vi "Activate Menu.vi"(7 "Coords":T1, 8 "error in":errorcluster, 9 "Menu Ref":refnum<k9>, 10 "Control Ref":refnum<vi>, 11 "Peer Review":refnum<class "Peer Review.lvclass">) -> (0 "error out":errorcluster, 2 "Discard?":bool)   [LabVIEW 2020, in "Peer Review.lvclass"]
uses:
  Peer Review.lvclass
  <vilib>/Utility/miscctls.llb/LVPoint32TypeDef.ctl
  Peer Review.lvclass/Peer Review.ctl
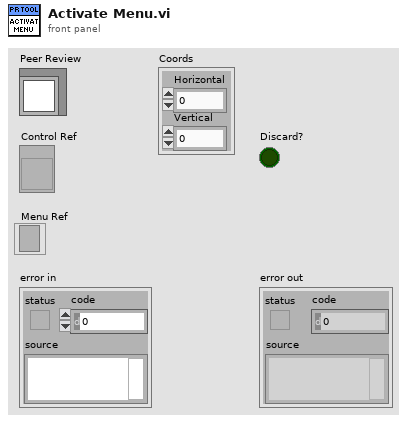
[diagram p1: front panel]
types:
  T1 = typedef "LVPoint32TypeDef.ctl" = cluster{"Horizontal":i32, "Vertical":i32}
  T2 = typedef "LVRowAndColumnTypeDef.ctl" = cluster{"Row":i32, "Column":i32}
  T3 = typedef "Peer Review.lvclass/File Info.ctl" = cluster{"File ID":i32, "Commit ID":i32, "Reviewed Hash":string, "Relative Path":string, "File Path":path, "File Checksum":string, "State":T4, "FP Changes":i32, "BD Changes":i32, "FP Bounds Error":dbl, "BD Bounds Error":dbl, "Lines Added":i32, "Lines Removed":i32, "Analysis Passes":i32, "Analysis Fails":i32, "Attribute Changes":i32, "Reentrancy Changes":string, "Cyclomatic Complexity":i32, "Node Count":i32, "Revision Number":u32, "LabVIEW Version":string, "Description":string, "Master Path":path, "Master Checksum":string, "VI Type":T5, "LabVIEW File":bool, "Review Complete":bool, "File Ref":refnum<vi>}
  T4 = typedef "Peer Review.lvclass/File State.ctl" = enum16{"Interrogation Needed", "Modified", "Deleted", "Added", "Matches Previous", "No Changes", "Moved"}
  T5 = typedef "Peer Review.lvclass/VI Type.ctl" = enum32{"invalid VI type", "Standard VI", "Control VI", "Global VI", "Polymorphic VI", "Configuration VI", "SubSystem", "Facade VI", "Method VI", "Statechart Diagram VI"}
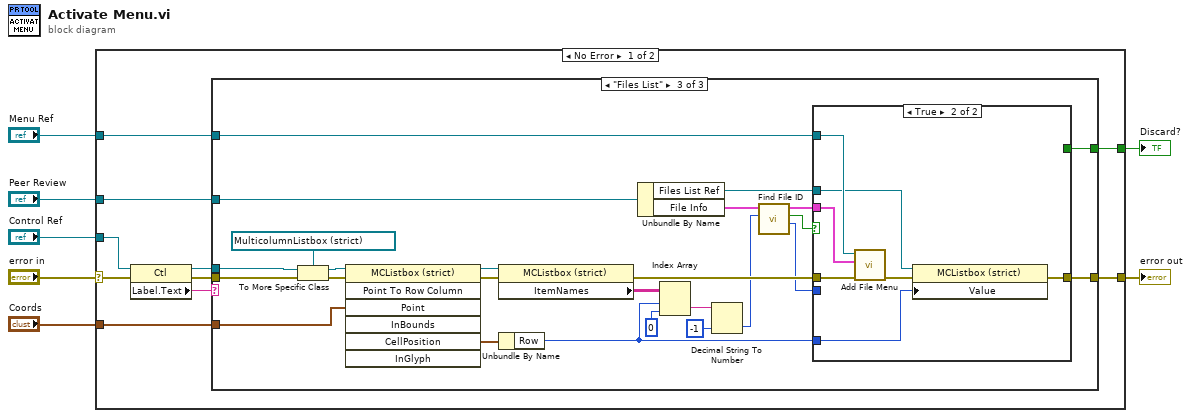
[diagram p0: block diagram]
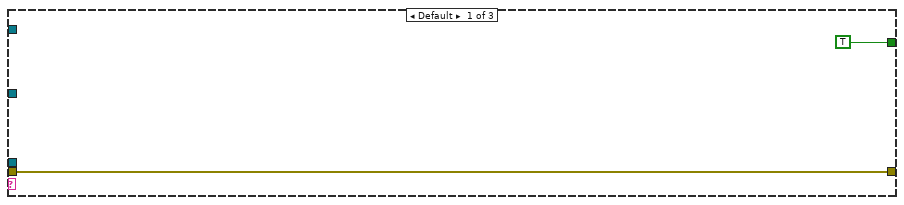
[diagram p2: hidden frame]
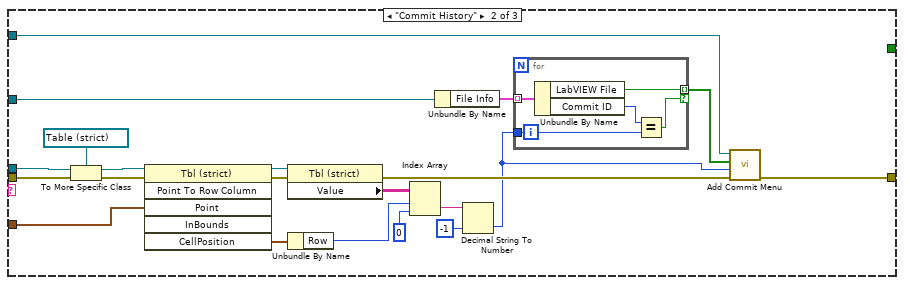
[diagram p3: hidden frame]
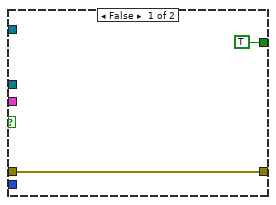
[diagram p4: hidden frame]
diagram:
  n1 = case shown="No Error" "error in" {
    selector: "error in" -> [w16 w80]
    tunnel: "Control Ref" -> [w17 _]
    tunnel: "Coords" -> [w13 _]
    tunnel: "Menu Ref" -> [w11 _]
    tunnel: [w10 w80] -> w3
    tunnel: [w9 _] -> w2
    tunnel: "Peer Review" -> [w8 _]
    frame No Error {
      n2 = property class="Ctl"(reference=w17, error in=w16) -> (reference out=w14:refnum<vi>, error out=w15:errorcluster, "Label.Text"=w12:string)
      n3 = case shown="\"Files List\"" w12 {
        tunnel: w15 -> [w19 w39 w70]
        tunnel: w14 -> [_ w38 w69]
        tunnel: w13 -> [_ w37 w68]
        tunnel: w11 -> [_ w34 w65]
        tunnel: [w19 w33 w64] -> w10
        tunnel: [TRUE _ w63] -> w9
        tunnel: w8 -> [_ w25 w55]
        frame Default {
        }
        frame "Commit History" {
          n4 = To More Specific Class(target class=refnum<vi> refnum ("Commit History Ref"), reference=w38, error in=w39) -> (specific class reference=w29:refnum<vi>, error out=w30:errorcluster)
          n5 = invoke class="Tbl (strict)" method="Point To Row Column"(reference=w29, error in=w30, "Point"=w37) -> (reference out=w27:refnum<vi>, error out=w26:errorcluster, "CellPosition"=w28:T2)  [unwired: 3 in, 3 out]
          n6 = property class="Tbl (strict)"(reference=w27, error in=w26) -> (error out=w35:errorcluster, "Value"=w36:string[][])  [unwired: 1 out]
          n7 = Unbundle By Name(w28) -> ("Row"=w40:i32)
          n8 = Index Array(array=w36, index (row)=w40, index (col)=0 ("disabled index (col)")) -> (element=w20:string)
          n9 = Unbundle By Name(w25) -> ("File Info"=w32:T3[])
          n10 = Decimal String To Number(string=w20, default (0L)=-1 ("default (0 I32)")) -> (number=w22:i32)  [unwired: 1 in, 1 out]
          n11 = for {
            tunnel: w32 -> [w44] mode=indexing
            tunnel: w22 -> [w45]
            tunnel: [w41] -> w23 mode=indexing if=w42
            n12 = Unbundle By Name(w44) -> ("LabVIEW File"=w41:bool, "Commit ID"=w43:i32)
            n13 = Equal?(x=w43, y=w45) -> (x = y?=w42:bool)
          }
          n14 = call "Add Commit Menu.vi"("error in"=w35, "Commit ID"=w22, "LabVIEW Files?"=w23, "Menu Ref"=w34) -> ("error out"=w33:errorcluster)  [unwired: 7 in]
        }
        frame "Files List" {
          n15 = To More Specific Class(target class=refnum<vi> refnum ("Files List Ref"), reference=w69, error in=w70) -> (specific class reference=w59:refnum<vi>, error out=w60:errorcluster)
          n16 = invoke class="MCListbox (strict)" method="Point To Row Column"(reference=w59, error in=w60, "Point"=w68) -> (reference out=w57:refnum<vi>, error out=w56:errorcluster, "CellPosition"=w58:T2)  [unwired: 4 in, 4 out]
          n17 = property class="MCListbox (strict)"(reference=w57, error in=w56) -> (error out=w66:errorcluster, "ItemNames"=w67:string[][])  [unwired: 1 out]
          n18 = Unbundle By Name(w58) -> ("Row"=w46:i32)
          n19 = Unbundle By Name(w55) -> ("Files List Ref"=w48:refnum<vi>, "File Info"=w52:T3[])
          n20 = Index Array(array=w67, index (row)=w46, index (col)=0 ("disabled index (col)")) -> (element=w53:string)
          n21 = Decimal String To Number(string=w53, default (0L)=-1 ("default (0 I32)")) -> (number=w51:i32)  [unwired: 1 in, 1 out]
          n22 = call "Find File ID.vi"("File ID"=w51, "File List"=w52) -> ("Array Index"=w47:i32, "Found?"=w50:bool, "File Info"=w49:T3)  [unwired: 7 in]
          n23 = case shown="True" w50 {
            tunnel: w66 -> [w72 w78]
            tunnel: w65 -> [_ w79]
            tunnel: [w72 w77] -> w64
            tunnel: [TRUE _] -> w63
            tunnel: w49 -> [_ w76]
            tunnel: w48 -> [_ w74]
            tunnel: w47 -> [_ _]
            tunnel: w46 -> [_ w75]
            frame False {
            }
            frame True {
              n24 = call "Add File Menu.vi"("error in"=w78, "File Info"=w76, "Menu Ref"=w79) -> ("error out"=w73:errorcluster)  [unwired: 8 in]
              n25 = property class="MCListbox (strict)"(reference=w74, error in=w73, "Value"=w75) -> (error out=w77:errorcluster)  [unwired: 1 out]
            }
          }
        }
      }
    }
    frame Error {
    }
  }
  "error out" <- w3
  "Discard?" <- w2
